vi "Do.vi"(8 "error in (no error)":errorcluster, 10 "Actor in":refnum<class "Actor.lvclass">, 11 "Set Delays Msg":refnum<class "Set Delays Msg.lvclass">) -> (0 "error out":errorcluster, 2 "Actor out":refnum<class "Actor.lvclass">)   [LabVIEW 2020, in "BNT_ULx.lvlib" / "Set Delays Msg.lvclass"]
doc: "This VI delivers the message to the actor by calling the appropriate method(s) on the actor."
uses:
  Set Delays Msg.lvclass
  <vilib>/ActorFramework/Actor/Actor.lvclass
  C:/User/Brand/LVP/CSPP/CSPP-Template/Packages/CSPP_Core/Messages/CSPP_PVUpdate Msg/CSPP_PVUpdate Msg.lvclass
  CSPP_Core/Messages/CSPP_PVUpdate Msg/CSPP_PVUpdate Msg.lvclass/CSPP_PVUpdate Msg.ctl
  CSPP_Core/Classes/CSPP_ProcessVariables/ProcessVariable/PV.lvclass/PV.ctl
  Set Delays Msg.lvclass/Set Delays Msg.ctl
  CSPP_Core/Classes/CSPP_ProcessVariables/ProcessVariable/PV.lvclass
  CSPP_Core/Messages/CSPP_PVUpdate Msg/CSPP_PVUpdate Msg.lvclass
  BNT_ULx-MCSV-DOPWM/BNT_ULx-MCSV-DOPWM.lvclass
  C:/User/Brand/LVP/CSPP/CSPP-Template/Packages/CSPP_Core/Messages/CSPP_AsyncCallbackMsg/CSPP_AsyncCallback Msg.lvclass
  C:/Program Files (x86)/National Instruments/LabVIEW 2020/vi.lib/ActorFramework/Message/Message.lvclass
  C:/User/Brand/LVP/CSPP/CSPP-Template/Packages/BNT_ULx/BNT_ULx-MCSV/BNT_ULx-MCSV-DOPWM Messages/Set Delays Msg/Set Delays Msg.lvclass
  C:/User/Brand/LVP/CSPP/CSPP-Template/Packages/BNT_ULx/BNT_ULx-MCSV/BNT_ULx-MCSV/BNT_ULx-MCSV.lvclass
  C:/User/Brand/LVP/CSPP/CSPP-Template/Packages/CSPP_Core/Actors/CSPP_DeviceActor/CSPP_DeviceActor.lvclass
  C:/User/Brand/LVP/CSPP/CSPP-Template/Packages/CSPP_Core/Actors/CSPP_BaseActor/CSPP_BaseActor.lvclass
  C:/Program Files (x86)/National Instruments/LabVIEW 2020/vi.lib/ActorFramework/Actor/Actor.lvclass
  C:/User/Brand/LVP/CSPP/CSPP-Template/Packages/BNT_ULx/BNT_ULx-MCSV/BNT_ULx-MCSV-DOPWM/BNT_ULx-MCSV-DOPWM.lvclass
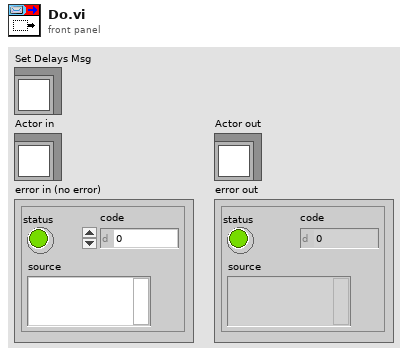
[diagram p1: front panel]
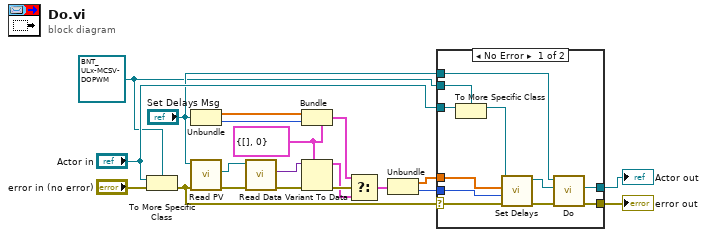
[diagram p0: block diagram]
diagram:
  w1 = refnum<class "BNT_ULx-MCSV-DOPWM.lvclass"> refnum ("BNT_ULx.lvlib:BNT_ULx-MCSV-DOPWM.lvclass")
  w14 = cluster{"PWM Delays":dbl[], "Start Index":i32} {"PWM Delays"=[], "Start Index"=0} ("Type")
  n1 = To More Specific Class(target class=w1, reference="Actor in", error in="error in (no error)") -> (error out=w11:errorcluster)  [unwired: 1 out]
  n2 = Unbundle ("Pre-Unbundler")("Set Delays Msg") -> (w3:dbl[], w2:i32)
  n3 = call "Read PV.vi"("error in (no error)"=w11, "CS++PVUpdate Msg in"="Set Delays Msg") -> ("error out"=w16:errorcluster, "PV"=w13:refnum<class "PV.lvclass">)  [unwired: 7 in, 1 out]
  n4 = call "Read Data.vi"("error in (no error)"=w16, "PV in"=w13) -> ("error out"=w7:errorcluster, "Data"=w6:variant)  [unwired: 7 in, 1 out]
  n5 = Bundle ("Pre-Bundler")(cluster=w14, "PWM Delays"=w3, "Start Index"=w2) -> (w8:cluster{"PWM Delays":dbl[], "Start Index":i32})
  n6 = Variant To Data(error in=w7, type=w14, Variant=w6) -> (data=w9:cluster{"PWM Delays":dbl[], "Start Index":i32}, error out=w15:errorcluster)
  n7 = Select ("MainSelect")(t=w8, s=w15, f=w9) -> (s? t:f=w12:cluster{"PWM Delays":dbl[], "Start Index":i32})
  n8 = Unbundle ("Main-Unbundler")(w12) -> ("PWM Delays"=w5:dbl[], "Start Index"=w4:i32)
  n9 = case shown="No Error" w11 {
    selector: w11 -> [w24 w33]
    tunnel: [w28 w33] -> w19
    tunnel: [w29 w32] -> w18
    tunnel: "Actor in" -> [w31 w32]
    tunnel: w1 -> [w30 _]
    tunnel: "Set Delays Msg" -> [w27 _]
    tunnel: w5 -> [w22 _]
    tunnel: w4 -> [w21 _]
    frame No Error {
      n10 = To More Specific Class ("To More Specific Class (internal)")(target class=w30, reference=w31) -> (specific class reference=w26:refnum<class "BNT_ULx-MCSV-DOPWM.lvclass">)  [unwired: 1 in, 1 out]
      n11 = call "Set Delays.vi"("error in"=w24, "Start Index"=w21, "PWM Delays"=w22, "BNT_ULx-MCSV-DOPWM in"=w26) -> ("error out"=w23:errorcluster, "BNT_ULx-MCSV-DOPWM out"=w25:refnum<class "BNT_ULx-MCSV-DOPWM.lvclass">)  [unwired: 6 in]
      n12 = call-parent "Do.vi"("error in (no error)"=w23, "Actor in"=w25, "CS++PVUpdate Msg"=w27) -> ("error out"=w28:errorcluster, "Actor out"=w29:refnum<class "Actor.lvclass">)  [unwired: 7 in]
    }
    frame Error {
    }
  }
  "error out" <- w19
  "Actor out" <- w18
